vi "log operation mode errors.vi"(8 "error in (no error)":errorcluster, 11 "Channel in":refnum<class "Channel.lvclass">) -> (0 "error out":errorcluster, 3 "Channel out":refnum<class "Channel.lvclass">)   [LabVIEW 2018, in "Channel.lvclass"]
uses:
  Channel.lvclass
  Channel.lvclass/Channel.ctl
  Sim_CCD/Sim_CCD.lvclass/Sim_CCD.ctl
  Sim_CCD/Sim_CCD.lvclass
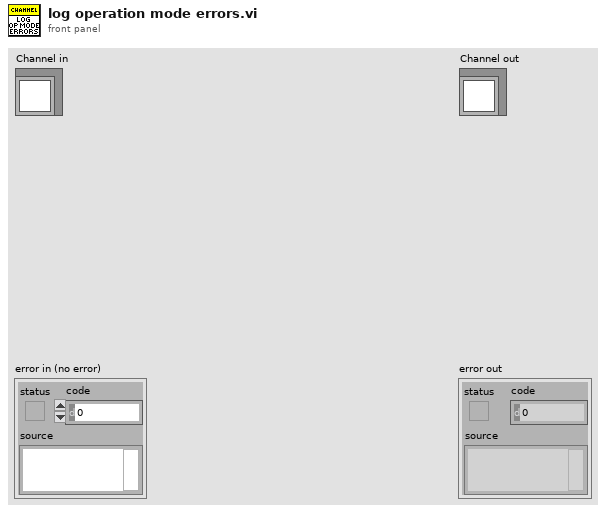
[diagram p1: front panel]
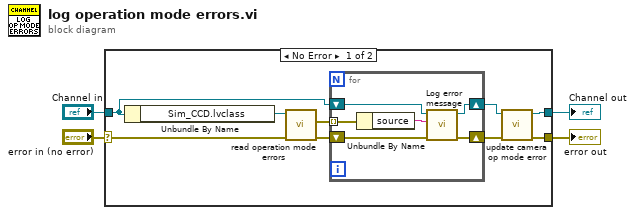
[diagram p0: block diagram]
diagram:
  n1 = case shown="No Error" "error in (no error)" {
    selector: "error in (no error)" -> [w10 w21]
    tunnel: [w7 w21] -> w3
    tunnel: [w5 w20] -> w1
    tunnel: "Channel in" -> [w6 w20]
    frame No Error {
      n2 = Unbundle By Name(w6) -> ("Sim_CCD.lvclass"=w11:refnum<class "Sim_CCD.lvclass">)
      n3 = call "read operation mode errors.vi"("error in (no error)"=w10, "Simulated_CCD_Camera in"=w11) -> ("error out"=w9:errorcluster, "WRITE SETUP errors"=w8:errorcluster[])  [unwired: 7 in, 1 out]
      n4 = for {
        shift-right: [w18] -> w12
        shift-left: w6 -> [w19]
        shift-right: [w17] -> w13
        shift-left: w9 -> [w16]
        tunnel: w8 -> [w14] mode=indexing
        n5 = Unbundle By Name(w14) -> ("source"=w15:string)
        n6 = call "Log error message.vi"("error in (no error)"=w16, "String"=w15, "Channel in"=w19) -> ("error out"=w17:errorcluster, "Channel out"=w18:refnum<class "Channel.lvclass">)  [unwired: 7 in]
      }
      n7 = call-dynamic "update camera op mode error.vi"("error in (no error)"=w13, "Channel in"=w12) -> ("error out"=w7:errorcluster, "Channel out"=w5:refnum<class "Channel.lvclass">)  [unwired: 8 in]
    }
    frame Error {
    }
  }
  "error out" <- w3
  "Channel out" <- w1
